vi "Clear Undo Flag.vi"(8 "error in":errorcluster, 11 "History in":refnum<class "History.lvclass">) -> (0 "error out":errorcluster, 3 "History out":refnum<class "History.lvclass">)   [LabVIEW 2020, in "lv_icon.lvlib" / "History.lvlib" / "History.lvclass"]
doc: "Clears an internal flag telling the History there is a state change to add to the undo stack."
uses:
  History.lvclass
  History.lvclass/History.ctl
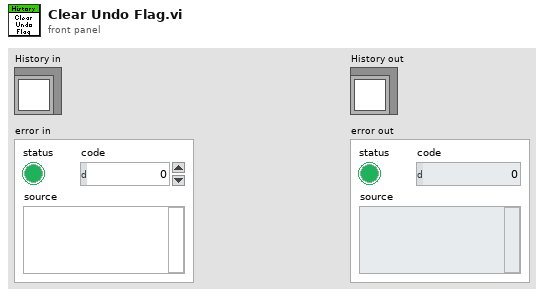
[diagram p1: front panel]
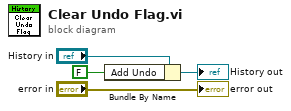
[diagram p0: block diagram]
diagram:
  n1 = Bundle By Name(cluster="History in", "Add Undo"=FALSE) -> (→"History out":refnum<class "History.lvclass">)
  "error out" <- "error in"
